vi "Raw Data Interpretor.vi"   [LabVIEW 2013]
doc: "Interpret raw sensor data by applying transformations and calibrations to it."
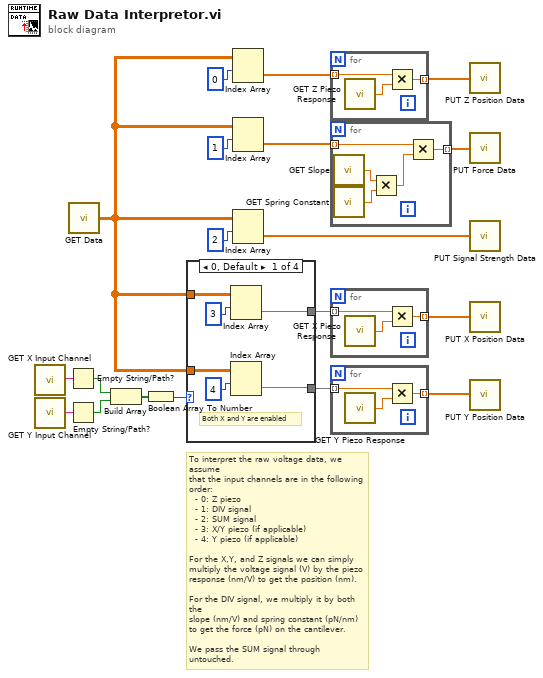
[diagram p0: block diagram]
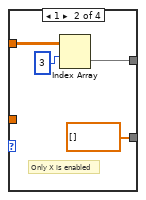
[diagram p2: hidden frame]
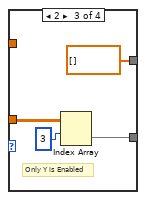
[diagram p3: hidden frame]
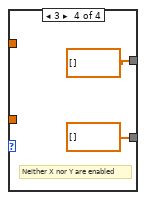
[diagram p4: hidden frame]
diagram:
  # "To interpret the raw voltage data, we assume\nthat the input channels are in the following\norder:\n  - 0: Z piezo\n  - 1: DIV signal\n  - 2: SUM signal\n  - 3: X/Y piezo (if applicable)\n  - 4: Y piezo (if applicable)\n\nFor the X,Y, and Z signals we can simply \nmultiply the voltage signal (V) by the piezo\nresponse (nm/V) to get the position (nm).\n\nFor the DIV signal, we multiply it by both the\nslope (nm/V) and spring constant (pN/nm)\nto get the force (pN) on the cantilever.\n\nWe pass the SUM signal through untouched."
  n1 = call "GET X Input Channel.vi"() -> ("X Input Channel"=w16:string)
  n2 = call "GET Y Input Channel.vi"() -> ("Y Input Channel"=w17:string)
  n3 = Empty String/Path?(string/path=w16) -> (empty?=w18:bool)
  n4 = Empty String/Path?(string/path=w17) -> (empty?=w15:bool)
  n5 = call "GET Data.vi"() -> ("Data"=w6:dbl[][])
  n6 = Build Array(w18, w15) -> (w19:bool[])
  n7 = Boolean Array To Number(Boolean array=w19) -> (number=w14:u32)
  n8 = case shown="0, Default" w14 {
    tunnel: w6 -> [w24 w28 _ _]
    tunnel: w6 -> [w22 _ w32 _]
    tunnel: [w20 dbl[] [] ("Sensor Data") w31 dbl[] [] ("Sensor Data")] -> w7
    tunnel: [w21 w27 dbl[] [] ("Sensor Data") dbl[] [] ("Sensor Data")] -> w8
    frame 0, Default {
      # "Both X and Y are enabled"
      n9 = Index Array(array=w24, index (row)=3) -> (element=w21:dbl[])  [unwired: 1 in]
      n10 = Index Array(array=w22, index (row)=4) -> (element=w20:dbl[])  [unwired: 1 in]
    }
    frame 1 {
      # "Only X is enabled"
      n11 = Index Array(array=w28, index (row)=3) -> (element=w27:dbl[])  [unwired: 1 in]
    }
    frame 2 {
      # "Only Y is Enabled"
      n12 = Index Array(array=w32, index (row)=3) -> (element=w31:dbl[])  [unwired: 1 in]
    }
    frame 3 {
      # "Neither X nor Y are enabled"
    }
  }
  n13 = Index Array(array=w6, index (row)=0) -> (element=w10:dbl[])  [unwired: 1 in]
  n14 = Index Array(array=w6, index (row)=1) -> (element=w9:dbl[])  [unwired: 1 in]
  n15 = Index Array(array=w6, index (row)=2) -> (element=w3:dbl[])  [unwired: 1 in]
  n16 = for {
    tunnel: w10 -> [w38] mode=indexing
    tunnel: [w36] -> w5 mode=indexing
    n17 = call "GET Z Piezo Response.vi"() -> ("Z Piezo Response"=w37:dbl)
    n18 = Multiply(x=w38, y=w37) -> (x*y=w36:dbl)
  }
  n19 = for {
    tunnel: w9 -> [w43] mode=indexing
    tunnel: [w42] -> w4 mode=indexing
    n20 = call "GET Slope.vi"() -> ("Slope"=w40:dbl)
    n21 = call "GET Spring Constant.vi"() -> ("Spring Constant"=w39:dbl)
    n22 = Multiply(x=w40, y=w39) -> (x*y=w41:dbl)
    n23 = Multiply(x=w43, y=w41) -> (x*y=w42:dbl)
  }
  n24 = for {
    tunnel: w8 -> [w46] mode=indexing
    tunnel: [w44] -> w2 mode=indexing
    n25 = call "GET X Piezo Response.vi"() -> ("X Piezo Response"=w45:dbl)
    n26 = Multiply(x=w46, y=w45) -> (x*y=w44:dbl)
  }
  n27 = for {
    tunnel: w7 -> [w49] mode=indexing
    tunnel: [w47] -> w1 mode=indexing
    n28 = call "GET Y Piezo Response.vi"() -> ("Y Piezo Response"=w48:dbl)
    n29 = Multiply(x=w49, y=w48) -> (x*y=w47:dbl)
  }
  n30 = call "PUT Z Position Data.vi"("Z Position Data"=w5) -> ()
  n31 = call "PUT Force Data.vi"("Force Data"=w4) -> ()
  n32 = call "PUT Signal Strength Data.vi"("Signal Strength Data"=w3) -> ()
  n33 = call "PUT X Position Data.vi"("X Position Data"=w2) -> ()
  n34 = call "PUT Y Position Data.vi"("Y Position Data"=w1) -> ()
